vi "Invertek Drive Params.vi"() -> ()   [LabVIEW 2020]
doc: "Modbus RTU for Invertek drives. Paul Nathan 19-JUN-2022."
panel:
  in  "max. freq. (Hz)":dbl[](array[numeric])=[0.0, 50.0, 50.0]
  in  "max. RPM (/min)":dbl[](array[numeric])=[0.0, 750.0, 750.0]
  in  "Serial timeout (ms)":u32=2000
  in  "Serial baud (bps)":u32=115200
  # "*max. RPM is the no-load synchronous RPM at 50 Hz full input. Generally this is:\nu_max (/min) = 60 * f_max * 2 / n_poles."
  # "max. RPM and max. freq values must match those in drive configuration P-01 either with P-10 set to zero or set to motor nameplate RPM. Max. freq. is determined by the mains supply infrastructure. In the UK it is 50 Hz."
  # "Serial baud rate must match the value in drive configuration P-36 index 2. This is particularly relevant if using a generic USB-RS485 converter. All network devices must have the same baud rate."
  # "Note that there is no drive address 0. Addresses start at 1. Array index and drive address have a 1:1 value correspondence."
  # "Drive addr."
  # "Drive addr."
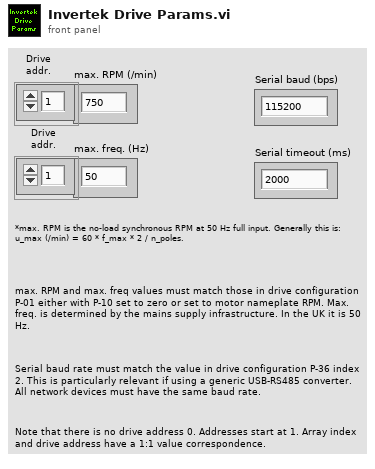
[diagram p1: front panel]
diagram:
